vi "adduser.vi"() -> ()   [LabVIEW 2012]
uses:
  <vilib>/Utility/file.llb/Read From Spreadsheet File (string).vi
panel:
  out "提示 2":string
  out "提示":string
  in  "确定":bool
  in  "psw":T1
  in  "username":T1
  in  "psw 2":T1
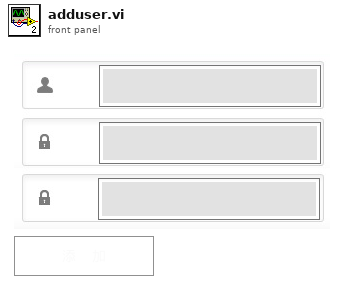
[diagram p1: front panel]
types:
  T1 = typedef "用户输入.ctl" = string
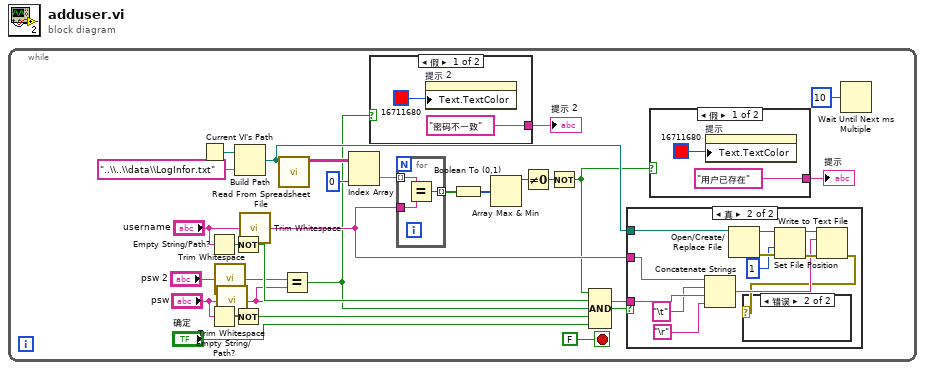
[diagram p0: block diagram]
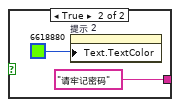
[diagram p2: hidden frame]
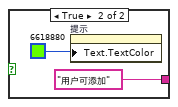
[diagram p3: hidden frame]
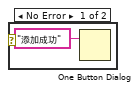
[diagram p5: hidden frame]
diagram:
  n1 = while {
    stop <- FALSE stop-if-true
    n2 = Current VI's Path() -> (path=w18:path)
    n3 = Empty String/Path?(string/path="username") -> (empty?=w25:bool)
    n4 = Empty String/Path?(string/path="psw") -> (empty?=w24:bool)
    n5 = call <vilib>:"Trim Whitespace.vi"("string"="psw 2") -> ("trimmed string"=w3:string)  [unwired: 1 in]
    n6 = call <vilib>:"Trim Whitespace.vi"("string"="psw") -> ("trimmed string"=w4:string)  [unwired: 1 in]
    n7 = Not(x=w25) -> (.not. x?=w22:bool)
    n8 = Not(x=w24) -> (.not. x?=w6:bool)
    n9 = Build Path(base path=w18, name or relative path="..\\..\\data\\LogInfor.txt" ("名称或相对路径")) -> (appended path=w17:path)
    n10 = call <vilib>:"Trim Whitespace.vi"("string"="username") -> ("trimmed string"=w15:string)  [unwired: 1 in]
    n11 = call-poly <vilib>:"Read From Spreadsheet File.vi"("file path (dialog if empty)"=w17) -> ("all rows"=w20:string[][])  [unwired: 6 in, 4 out]
    n12 = Equal?(x=w3, y=w4) -> (x = y?=w2:bool)
    n13 = Index Array(array=w20, index (col)=0 ("禁用的索引 (列)")) -> (element=w16:string[])  [unwired: 1 in]
    n14 = case shown="假" w2 {
      tunnel: ["密码不一致" "请牢记密码"] -> w1
      frame False {
        n15 = property on="提示 2" class="Str"("Text.TextColor"=u32 16711680 ("颜色盒")) -> ()  [unwired: 2 in, 2 out]
      }
      frame True {
        n16 = property on="提示 2" class="Str"("Text.TextColor"=u32 6618880 ("颜色盒")) -> ()  [unwired: 2 in, 2 out]
      }
    }
    "提示 2" <- w1
    n17 = for {
      tunnel: w16 -> [w39] mode=indexing
      tunnel: w15 -> [w38]
      tunnel: [w37] -> w14 mode=indexing
      n18 = Equal?(x=w39, y=w38) -> (x = y?=w37:bool)
    }
    n19 = Boolean To (0,1)(Boolean=w14) -> (0, 1=w13:i16[])
    n20 = Array Max & Min(array=w13) -> (max value=w12:i16)  [unwired: 3 out]
    n21 = Not Equal To 0?(x=w12) -> (x != 0?=w11:bool)
    n22 = Not(x=w11) -> (.not. x?=w8:bool)
    n23 = Compound Arithmetic op=AND(w8, w22, w2, w6, "确定") -> (w23:bool)
    n24 = case shown="真" w23 {
      tunnel: w4 -> [_ w45]
      tunnel: w15 -> [_ w51]
      tunnel: w17 -> [_ w41]
      frame False {
      }
      frame True {
        n25 = Concatenate Strings(w51, "\t", w45, "\r") -> (w43:string)
        n26 = Open/Create/Replace File(file path (use dialog)=w41) -> (refnum out=w48:refnum<file>, error out=w47:errorcluster)  [unwired: 5 in, 1 out]
        n27 = Set File Position(refnum=w48, from (0:start)=1, error in=w47) -> (refnum out=w49:refnum<file>, error out=w50:errorcluster)  [unwired: 1 in]
        n28 = Write to Text File(file (use dialog)=w49, text=w43, error in=w50) -> (error out=w40:errorcluster)  [unwired: 1 in, 2 out]
        n29 = case shown="错误" w40 {
          frame No Error {
            n30 = One Button Dialog(message="添加成功" ("消息")) -> ()  [unwired: 1 in, 1 out]
          }
          frame Error {
          }
        }
      }
    }
    n31 = case shown="假" w8 {
      tunnel: ["用户已存在" "用户可添加"] -> w9
      frame False {
        n32 = property on="提示" class="Str"("Text.TextColor"=u32 16711680 ("颜色盒")) -> ()  [unwired: 2 in, 2 out]
      }
      frame True {
        n33 = property on="提示" class="Str"("Text.TextColor"=u32 6618880 ("颜色盒")) -> ()  [unwired: 2 in, 2 out]
      }
    }
    "提示" <- w9
    n34 = Wait Until Next ms Multiple(millisecond multiple=u32 10 ("毫秒倍数")) -> ()  [unwired: 1 out]
  }
